vi "ief_get_axis_parameter_min.vi"(3 "error in (no error)":errorcluster, 4 "Axis Parameter":u16(ring) items=["drving speed", "reference speed", "manual speed", "slow motion speed", "start-stop speed", "acceleration", "gear factor", "driving range minimum", "driving range maximum", "motor phase current", "motor sleep current", "P-share", "I-share", "D-share", "encoder pulses per revolution", "position window", "maximum error", "range of end switches", "effectiv revolution", "P-current regulator", "I-current regulator", "regulator type", "sequence of reference run", "revolution direction", "revolution monitoring activated", "steps per revolution", "full-steps per revolution", "axis end switch changed", "display unit", "ramp type", "invert rotary encoder direction", "end switch type", "distance between 0 and reference switch", "rotary encoder synchronisation", "adopt rotary encoder position", "activate break in measurement mode", "activate absolute positioning system", "APS transmission frequency divider", "APS delay time divider", "APS evaluation code", "APS multiturn", "APS number of SSI databits", "APS bit 25 function", "APS feed rate", "APS reference point offset", "invert direction", "APS inkrement per revolution", "APS maximum revolution number", "APS position evaluation databit number"], 5 "Axis Number":u16=1 min=1 max=16, 6 "Tagprefix in":refnum<k21>) -> (0 "error out (no error)":errorcluster, 1 "Parameter Value":sgl format="%.2f", 2 "Tagprefix out":refnum<k21>)   [LabVIEW 2015, in "IEF Werner.lvlib"]
doc: "The VI reads the present minimum value of the specified axis parameter of the chosen axis.\n\nAxis Range:\n01 - 10 hex\n1 - 16 dec\n\nAxis Parameter Range:\n01 hex, 1 dec - driving speed\n02 hex, 2 dec - reference speed\n03 hex, 3 dec - manual speed\n04 hex, 4 dec - slow motion speed\n05 hex, 5 dec - start-stop speed\n06 hex, 6 dec - acceleration\n07 hex, 7 dec - gear factor\n08 hex, 8 dec - driving range minimum\n09 hex, 9 dec - driving range maximum\n0A hex, 10 dec - motor phase current\n0B hex, 11 dec - motor sleep current\n0C hex, 12 dec - P-share\n0D hex, 13 dec - I-share\n0E hex, 14 dec - D-share\n0F hex, 15 dec - encoder pulses per revolution\n10 hex, 16 dec - position window\n11 hex, 17 dec - maximum error\n12 hex, 18 dec - range of end switches \n13 hex, 19 dec - effective revolution\n14 hex, 20 dec - P-current regulator\n15 hex, 21 dec - I-current regulator\n16 hex, 22 dec - regulator type\n17 hex, 23 dec - sequence of reference run\n18 hex, 24 dec - revolution direction\n19 hex, 25 dec - revolution monitoring activated\n1A hex, 26 dec - steps per revolution\n1B hex, 27 dec - full-steps per revolution\n1C hex, 28 dec - axis end switch changed\n1D hex, 29 dec - display unit\n1Ehex, 30 dec - ramp type\n1F hex, 31 dec - invert rotary encoder direction\n20 hex, 32 dec - end switch type\n21 hex, 33 dec - distance between 0 and reference switch\n22 hex, 34 dec - rotary encoder synchronisation\n23 hex, 35 dec - adopt rotary encoder position\n24 hex, 36 dec - activate break in measurement mode\n25 hex, 37 dec - activate absolute positioning system\n26 hex, 38 dec - APS transmission frequency divider\n27 hex, 39 dec - APS delay time divider\n28 hex, 40 dec - APS evaluation code\n29 hex, 41 dec - APS multiturn\n2A hex, 42 dec - APS number of SSI databits\n2B hex, 43 dec - APS bit 25 function\n2C hex, 44 dec - APS feed rate\n2D hex, 45 dec - APS reference point offset\n2E hex, 46 dec - APS invert direction\n2F hex, 47 dec - APS inkrement per revolution\n30 hex, 48 dec - APS maximum revolution number\n31 hex, 49 dec - APS position evaluation databit number"
uses:
  IEF Werner.lvlib
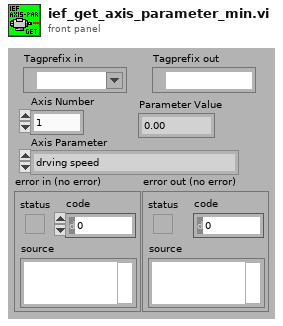
[diagram p1: front panel]
types:
  T1 = typedef "Semaphore RefNum" = refnum<k1>
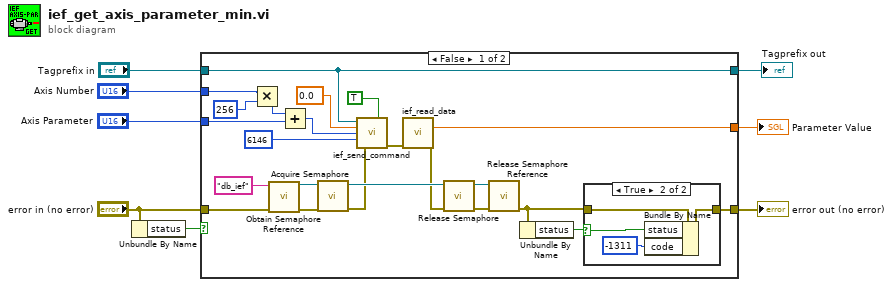
[diagram p0: block diagram]
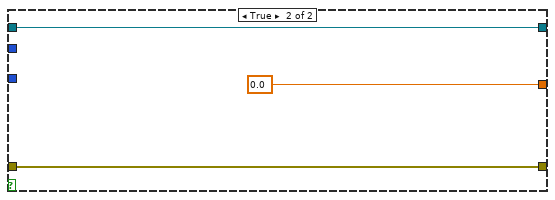
[diagram p3: hidden frame]
diagram:
  n1 = Unbundle By Name("error in (no error)") -> ("status"=w3:bool)
  n2 = case shown="False" w3 {
    tunnel: "error in (no error)" -> [w11 w39]
    tunnel: "Axis Number" -> [w29 _]
    tunnel: "Axis Parameter" -> [w27 _]
    tunnel: [w22 w39] -> w6
    tunnel: [w23 sgl 0.0 ("value real 32")] -> w5
    tunnel: "Tagprefix in" -> [w9 w38]
    tunnel: [w9 w38] -> w1
    frame False {
      n3 = Multiply(x=w29, y=u16 256) -> (x*y=w26:u16)
      n4 = call <vilib>:"Obtain Semaphore Reference.vi"("error in (no error)"=w11, "name (unnamed)"="db_ief") -> ("error out"=w18:errorcluster, "semaphore"=w17:T1)  [unwired: 3 in, 1 out]
      n5 = Add(x=w26, y=w27) -> (x+y=w25:u16)
      n6 = call <vilib>:"Acquire Semaphore.vi"("error in (no error)"=w18, "semaphore"=w17) -> ("error out"=w15:errorcluster, "semaphore out"=w19:T1)  [unwired: 3 in, 1 out]
      n7 = call "ief_send_command.vi"("Tagprefix in"=w9, "Command datum of type real"=TRUE, "Command datum"=sgl 0.0, "Command parameter"=w25, "Command code"=u16 6146, "error in (no error)"=w15) -> ("error out (no error)"=w24:errorcluster)  [unwired: 4 in, 5 out]
      n8 = call "ief_read_data.vi"("error in (no error)"=w24) -> ("value real 32"=w23:sgl, "error out (no error)"=w14:errorcluster)  [unwired: 8 in, 5 out]
      n9 = call <vilib>:"Release Semaphore.vi"("error in (no error)"=w14, "semaphore"=w19) -> ("error out"=w20:errorcluster, "semaphore out"=w21:T1)  [unwired: 4 in]
      n10 = call <vilib>:"Release Semaphore Reference.vi"("error in (no error)"=w20, "semaphore"=w21) -> ("error out"=w13:errorcluster)  [unwired: 8 in, 1 out]
      n11 = Unbundle By Name(w13) -> ("status"=w12:bool)
      n12 = case shown="True" w12 {
        selector: w12 -> [_ w33]
        tunnel: [w32 w36] -> w22
        tunnel: w13 -> [w32 w35]
        frame False {
        }
        frame True {
          n13 = Bundle By Name(cluster=w35, "status"=w33, "code"=-1311) -> (w36:errorcluster)
        }
      }
    }
    frame True {
    }
  }
  "error out (no error)" <- w6
  "Parameter Value" <- w5
  "Tagprefix out" <- w1
